vi "Setup.vi"(0 "levels file path":string, 1 "timing file path":string, 2 "specifications file path":string, 3 "pin map file path":string, 4 "resource name":string) -> (7 "instrument handle out":refnum<k15>, 10 "error out":errorcluster)   [LabVIEW 2018]
uses:
  <instrlib>/niDigital/niDigital.llb/niDigital Load Specifications Levels and Timing (Multiple).vi
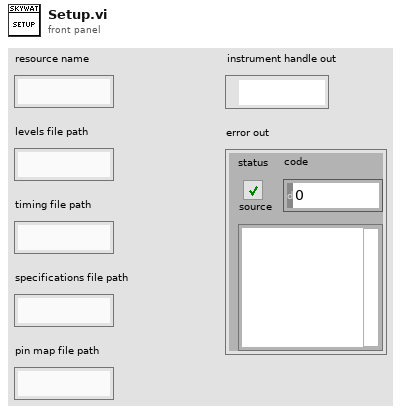
[diagram p1: front panel]
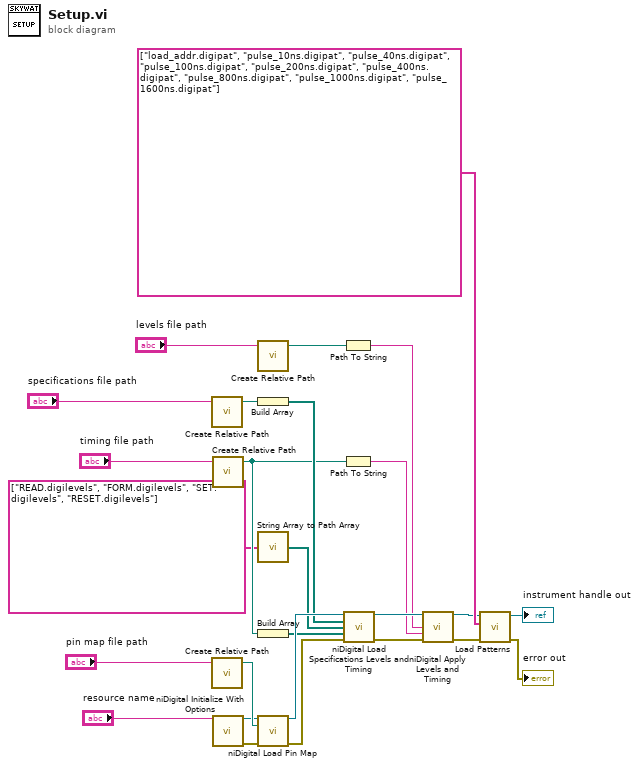
[diagram p0: block diagram]
diagram:
  n1 = call "Create Relative Path.vi"("file name"="specifications file path") -> ("appended path"=w6:path)  [unwired: 4 in]
  n2 = call "Create Relative Path.vi"("file name"="pin map file path") -> ("appended path"=w15:path)  [unwired: 4 in]
  n3 = call "Create Relative Path.vi"("file name"="timing file path") -> ("appended path"=w5:path)  [unwired: 4 in]
  n4 = call <instrlib>:"niDigital Initialize With Options.vi"("resource name"="resource name") -> ("instrument handle"=w13:refnum<k15>, "error out"=w14:errorcluster)  [unwired: 13 in]
  n5 = call "Create Relative Path.vi"("file name"="levels file path") -> ("appended path"=w3:path)  [unwired: 4 in]
  n6 = Build Array(w6) -> (w7:path[])
  n7 = call "String Array to Path Array.vi"("Array in"=string[] ["READ.digilevels", "FORM.digilevels", "SET.digilevels", "RESET.digilevels"]) -> ("Array out"=w1:path[])
  n8 = Build Array(w5) -> (w4:path[])
  n9 = call <instrlib>:"niDigital Load Pin Map.vi"("instrument handle"=w13, "pin map file"=w15, "error in"=w14) -> ("instrument handle out"=w25:refnum<k15>, "error out"=w26:errorcluster)  [unwired: 11 in]
  n10 = Path To String(path=w3) -> (string=w19:string)
  n11 = Path To String(path=w5) -> (string=w18:string)
  n12 = call-poly <instrlib>:"niDigital Load Specifications Levels and Timing.vi"("instrument handle"=w25, "specifications file paths"=w7, "levels file paths"=w1, "timing file paths"=w4, "error in"=w26) -> ("instrument handle out"=w23:refnum<k15>, "error out"=w22:errorcluster)  [unwired: 9 in]
  n13 = call <instrlib>:"niDigital Apply Levels and Timing.vi"("instrument handle"=w23, "levels sheet"=w19, "timing sheet"=w18, "error in"=w22) -> ("instrument handle out"=w9:refnum<k15>, "error out"=w8:errorcluster)  [unwired: 10 in]
  n14 = call "Load Patterns.vi"("error in (no error)"=w8, "patterns"=string[] ["load_addr.digipat", "pulse_10ns.digipat", "pulse_40ns.digipat", "pulse_100ns.digipat", "pulse_200ns.digipat", "pulse_400ns.digipat", "pulse_800ns.digipat", "pulse_1000ns.digipat", "pulse_1600ns.digipat"], "instrument handle"=w9) -> ("error out"=→"error out":errorcluster, "instrument handle out"=→"instrument handle out":refnum<k15>)  [unwired: 7 in]
